vi "PH_PILS.ExtShutters.vi"(0 "i ref in":refnum<vi>, 5 "error IO":errorcluster) -> (14 "i ref out":refnum<vi>, 19 "error out":errorcluster)   [LabVIEW 2014, in "PH_PILS.lvlib"]
doc: "This is the proc case \"_Boolean\"."
uses:
  PH_PILS.lvlib
  PH_Basics/PH_Common/PH_Common.lvlib
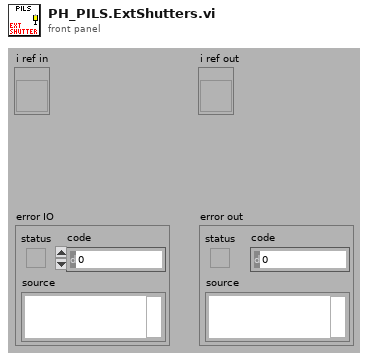
[diagram p1: front panel]
types:
  T1 = typedef "PH_PILS.lvlib/PH_PILS.i attribute.ctl" = cluster{"Boolean":cluster{"GUI Ref":refnum<vi>, "Status":i32}[], "GUI Refs Exp. Shutters":cluster{"1":refnum<vi>, "2":refnum<vi>, "3":refnum<vi>, "4":refnum<vi>}, "Tristate2Run GUI Refs":refnum<vi>[], "EO-Likes":cluster{"GUI Ref":refnum<vi>, "Status":i32}[], "Operation Mode":cluster{"Operation Mode":T2, "GUI":cluster{"Ref State":refnum<vi>, "Ref":refnum<vi>}, "Servicemode":cluster{"Tagname":string, "Status":i32}, "Labormode":cluster{"Tagname":string, "Status":i32}, "Searchmode":cluster{"Tagname":string, "Status":i32}, "Shotmode":cluster{"Tagname":string, "Status":i32}}, "Submode":cluster{"Submode":T3, "GUI":cluster{"Ref State":refnum<vi>, "Ref":refnum<vi>}, "Submode":cluster{"Tagname":string, "Status":i32}}, "Experiment":cluster{"Experiment":enum16{"unknown", "intern", "4 (Z6)", "3", "2", "1"}, "GUI":cluster{"Ref State":refnum<vi>, "Ref":refnum<vi>}, "intern":cluster{"Tagname":string, "Status":i32}, "Exp 4":cluster{"Tagname":string, "Status":i32}, "Exp 3":cluster{"Tagname":string, "Status":i32}, "Exp 2":cluster{"Tagname":string, "Status":i32}, "Exp 1":cluster{"Tagname":string, "Status":i32}}, "TristateNormal":cluster{"GUI Ref":refnum<vi>, "Status":i32}[], "Door Tags":cluster{"GUI Ref":refnum<vi>, "Status":i32}[], "GUIlessTags":cluster{"Name":string, "Status":i32}[], "Beamline GUI Refs":refnum<vi>[], "Special Boolean":cluster{"GUI Ref":refnum<vi>, "Status":i32}[], "Laserpower":cluster{"GUI Ref":refnum<vi>, "Status":i32}[], "Shutter":cluster{"GUI Ref":refnum<vi>, "Status":i32}[], "Tristate EO Like":cluster{"GUI Ref":refnum<vi>, "Status":i32}[], "PP":cluster{"GUI Ref":refnum<vi>, "Status":i32, "Head Ref":refnum<vi>, "Slider Ref":refnum<vi>}[], "Switch Knobs":cluster{"GUI Ref":refnum<vi>, "Status":i32}[], "Latch Knob GUI Refs":refnum<vi>[], "FailureCounter":i32, "Enabled Status":cluster{"Laser":i32, "PreAmp":i32, "MainAmp":i32}, "Mercury":refnum<vi>, "Instance Rods":string, "Logfile":path, "Beckhoff-Instance Internal":string, "Beckhoff-Instance External":string, "Enabling Rights":cluster{"Name":string, "Password":string, "PA?":bool, "MA?":bool, "Exp?":bool}[]}
  T2 = typedef "PH_PILS.lvlib/PH_PILS.Operation Mode.ctl" = enum16{"unknown", "Service", "Labor", "Search", "Shot"}
  T3 = typedef "PH_PILS.lvlib/PH_PILS.Submode.ctl" = enum16{"unknown", "HV-Normal", "HV-Test"}
  T4 = cluster{"1":refnum<vi>, "2":refnum<vi>, "3":refnum<vi>, "4":refnum<vi>}
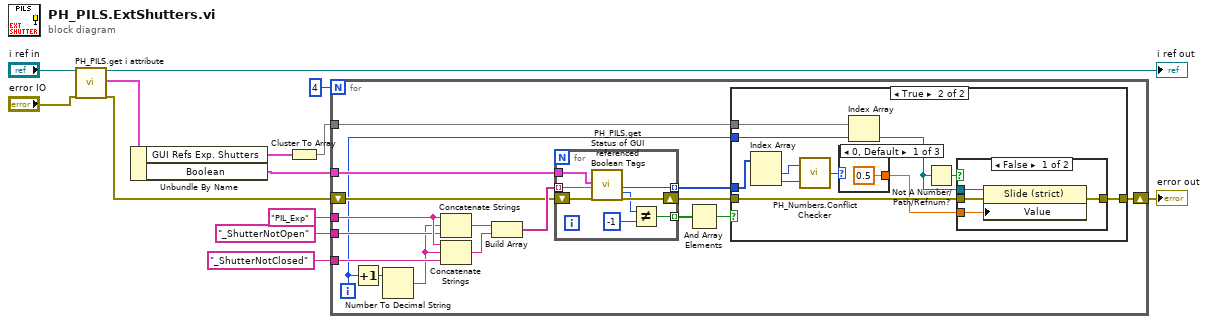
[diagram p0: block diagram]
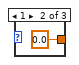
[diagram p3: hidden frame]
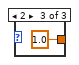
[diagram p4: hidden frame]
diagram:
  n1 = call "PH_PILS.get i attribute.vi"("i ref in"="i ref in", "error in (no error)"="error IO") -> ("i ref out"=→"i ref out":refnum<vi>, "i attribute"=w5:T1, "error out"=w6:errorcluster)  [unwired: 15 in]
  n2 = Unbundle By Name(w5) -> ("GUI Refs Exp. Shutters"=w4:T4, "Boolean"=w7:cluster{"GUI Ref":refnum<vi>, "Status":i32}[])
  n3 = Cluster To Array(cluster=w4) -> (array=w3:refnum<vi>[])
  n4 = for {
    N: 4 -> [_]
    tunnel: "PIL_Exp" -> [w30]
    tunnel: "_ShutterNotOpen" -> [w27]
    tunnel: "_ShutterNotClosed" -> [w29]
    tunnel: w7 -> [w22]
    shift-right: [w18] -> w2
    shift-left: w6 -> [w21]
    tunnel: w3 -> [w15]
    i -> [w14]
    n5 = Increment(x=w14) -> (x+1=w28:i32)
    n6 = Number To Decimal String(number=w28) -> (decimal integer string=w26:string)  [unwired: 1 in]
    n7 = Concatenate Strings(w30, w26, w27) -> (w24:string)
    n8 = Concatenate Strings(w30, w26, w29) -> (w25:string)
    n9 = Build Array(w24, w25) -> (w23:string[])
    n10 = for {
      tunnel: w23 -> [w58] mode=indexing
      shift-right: [w57] -> w19
      shift-left: w21 -> [w56]
      tunnel: w22 -> [w55]
      tunnel: [w54] -> w17 mode=indexing
      tunnel: [w51] -> w20 mode=indexing
      n11 = call "PH_PILS.get Status of GUI referenced Boolean Tags.vi"("Tags"=w55, "Tagname"=w58, "error in"=w56) -> ("Status"=w54:i32, "index of element"=w52:i32, "error out"=w57:errorcluster)  [unwired: 13 in, 1 out]
      n12 = Not Equal?(x=w52, y=-1 ("index of element")) -> (x != y?=w51:bool)
    }
    n13 = And Array Elements(Boolean array=w20) -> (logical AND=w16:bool)
    n14 = case shown="True" w16 {
      tunnel: w19 -> [w31 w41]
      tunnel: [w31 w40] -> w18
      tunnel: w17 -> [_ w39]
      tunnel: w15 -> [_ w33]
      tunnel: w14 -> [_ w32]
      frame False {
      }
      frame True {
        n15 = Index Array(array=w39) -> (element #1=w38:i32, element #2=w37:i32)  [unwired: 2 in]
        n16 = call "PH_Numbers.Conflict Checker.vi"("Input 2"=w37, "Input 1"=w38) -> ("Result"=w36:i32)
        n17 = case shown="0, Default" w36 {
          tunnel: [0.5 ("Value") 0.0 ("Value") 1.0 ("Value")] -> w35
          frame 0, Default {
          }
          frame 1 {
          }
          frame 2 {
          }
        }
        n18 = Index Array(array=w33, index=w32) -> (element=w34:refnum<vi>)
        n19 = Not A Number/Path/Refnum?(number/path/refnum=w34) -> (NaN/Path/Refnum?=w42:bool)
        n20 = case shown="False" w42 {
          tunnel: w34 -> [w49 _]
          tunnel: w41 -> [w48 w50]
          tunnel: [w47 w50] -> w40
          tunnel: w35 -> [w46 _]
          frame False {
            n21 = property class="Slide (strict)"(reference=w49, error in=w48, "Value"=w46) -> (error out=w47:errorcluster)  [unwired: 1 out]
          }
          frame True {
          }
        }
      }
    }
  }
  "error out" <- w2
